vi "LVCAM Nest Destroyed.vi"(10 "Nest Actor":refnum<class "LVCAM.lvclass">, 11 "Process in":refnum<class "Process.lvclass">) -> (0 "error out":errorcluster, 3 "Process out":refnum<class "Process.lvclass">)   [LabVIEW 2021, in "Process.lvlib" / "Process.lvclass"]
uses:
  Process.lvclass
  LVCAM/LVCAM/LVCAM/LVCAM.lvclass
  Process.lvclass/Process.ctl
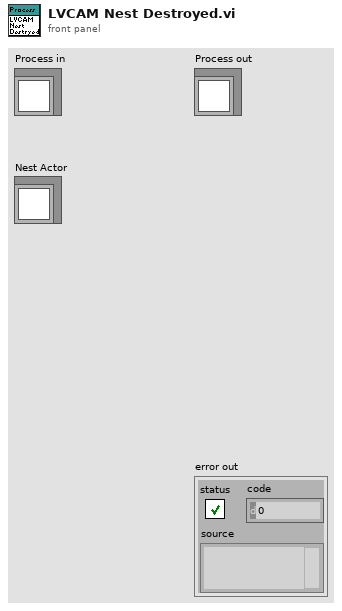
[diagram p1: front panel]
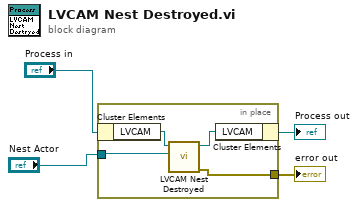
[diagram p0: block diagram]
diagram:
  n1 = in-place {
    in-place-border: "Nest Actor" -> [w6]
    in-place-border: [w5] -> w1
    n2 = in-place-cluster #1("Process in") -> ("LVCAM"=w8:refnum<class "LVCAM.lvclass">)
    n3 = call-dynamic "LVCAM Nest Destroyed.vi"("Nest Actor"=w6, "LVCAM Nest Destroyed in"=w8) -> ("error out"=w5:errorcluster, "LVCAM Nest Destroyed out"=w7:refnum<class "LVCAM.lvclass">)  [unwired: 8 in]
    n4 = in-place-cluster #1("LVCAM"=w7) -> (→"Process out":refnum<class "Process.lvclass">)
  }
  "error out" <- w1
